vi "Open.vi"(8 "error in (no error)":errorcluster, 11 "TcpClient in":refnum<class "TcpClient.lvclass">) -> (0 "error out":errorcluster, 3 "TcpClient out":refnum<class "TcpClient.lvclass">)   [LabVIEW 2021, in "TcpClient.lvlib" / "TcpClient.lvclass"]
uses:
  TcpClient.lvclass
  D:/_uliarczj/LabVIEW/LvTcpSocket/Source/TcpSocket/TcpSocket/TcpSocket.lvclass
  TcpSocket/TcpSocket/TcpSocket.lvclass/TcpSocket.ctl
  TcpSocket/TcpSocket/Read Address.vi
  TcpSocket/TcpSocket/Read Port.vi
  TcpSocket/TcpSocket/Read OpenTimeout.vi
  TcpSocket/TcpSocket/Write Connection.vi
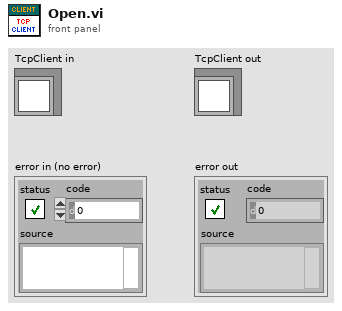
[diagram p1: front panel]
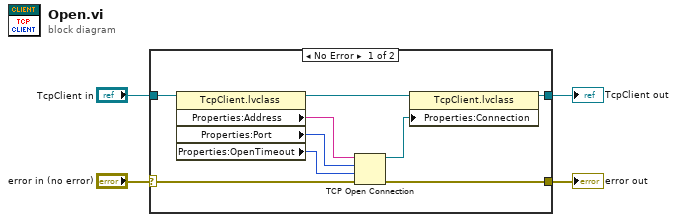
[diagram p0: block diagram]
diagram:
  n1 = case shown="No Error" "error in (no error)" {
    selector: "error in (no error)" -> [w13 w15]
    tunnel: [w12 w15] -> w3
    tunnel: [w9 w14] -> w2
    tunnel: "TcpClient in" -> [w11 w14]
    frame No Error {
      n2 = property class="TcpClient.lvclass"(reference=w11) -> (reference out=w10:refnum<class "TcpClient.lvclass">, "Properties:Address"=w8:string, "Properties:Port"=w7:u16, "Properties:OpenTimeout"=w6:i32)  [unwired: 1 in, 1 out]
      n3 = TCP Open Connection(address=w8, remote port or service name=w7, timeout ms (60000)=w6, error in (no error)=w13) -> (connection ID=w5:refnum<k5>, error out=w12:errorcluster)  [unwired: 1 in]
      n4 = property class="TcpClient.lvclass"(reference=w10, "Properties:Connection"=w5) -> (reference out=w9:refnum<class "TcpClient.lvclass">)  [unwired: 1 in, 1 out]
    }
    frame Error {
    }
  }
  "error out" <- w3
  "TcpClient out" <- w2
